vi "test_TxUDP.vi"() -> ()   [LabVIEW 2020]
uses:
  <instrlib>/AIM GmbH/_AIM 664/_controls/port_configuration.ctl
  <instrlib>/AIM GmbH/_AIM 664/_controls/port_speed.ctl
  <instrlib>/AIM GmbH/_AIM 664/_controls/comm_config_vl_tx.ctl
  <instrlib>/AIM GmbH/_AIM 664/_controls/comm_udp_tx.ctl
  <instrlib>/AIM GmbH/_AIM 664/helpers/EthFrameManagement/controls/arinc664_mac_src_info.ctl
  <instrlib>/AIM GmbH/_AIM 664/_controls/comm_computedMAC-IP.ctl
  <instrlib>/AIM GmbH/_AIM 664/bsp/Fdx Create Session (Tx-UDP Port-Oriented).vi
  <instrlib>/AIM GmbH/_AIM 664/bsp/Transmit/FdxCreateTxVL.vi
  <instrlib>/AIM GmbH/_AIM 664/bsp/Fdx Create UDP Port (TX-CommPort).vi
  <instrlib>/AIM GmbH/_AIM 664/bsp/Fdx Start (Tx).vi
  Global 1.vi
  <instrlib>/AIM GmbH/_AIM 664/bsp/Fdx Stop (Tx).vi
  <instrlib>/AIM GmbH/_AIM 664/AIM664LV.lvlib
  <instrlib>/AIM GmbH/_AIM 664/bsp/Fdx Create Session (Generic-Board).vi
  <instrlib>/AIM GmbH/_AIM 664/helpers/EthFrameManagement/EthFrameManagement.lvlib
panel:
  in  "index":i32
  out "Waveform Chart":u32(graph)
  out "CurrentIndex":u32
  out "IndexCycleCount":u32
  out "MsgCount":u32
  out "TxStatus":T1 {"TransmitMode" items=["FDX_TX_GENERIC", "FDX_TX_REPLAY", "FDX_TX_INDIVIDUAL"]; "TxStatus" items=["FDX_STAT_STOP", "FDX_STAT_RUN", "FDX_STAT_ERROR", "FDX_STAT_WAIT_F_TRIG"]}
  out "BytesWritten":u32
  in  "stop":bool
  out "IP configs":T2[](array[typedef]) {"MACsrc" format="%.0x"}
  out "Buf":u8[](array[numeric]) format="%.0x"
  in  "Buf Lenght":i32=512
  in  "VlTx":T3={"domainID"=1, "sideID"=1, "locationID"=1, "interfaceID"=1}
  in  "CommPort Config":T4[](array[typedef])=[{"PortType"=enum."FDX_UDP_SAMPLING", "partitionID"=1, "SubVlId"=1, "UdpSrcPort"=24, "UdpDstPort"=23, "SampleRateMs"=64.0, "UdpNumBufMessages"=1, "UdpMaxMessageSize"=512}]
  in  "VL Config":T5={"VlId"=60, "NumOfSubVl"=1, "rate ms [Bag]"=64, "domainID"=1, "sideID"=1, "locationID"=1, "interfaceID"=1, "NetSelect"=3, "Skew"=0, "MaxFrameLength"=1518, "FrameBufferSize"=0} {"NetSelect" items=["FDX_TX_FRAME_DLY_A"=0, "FDX_TX_FRAME_DLY_B"=1, "FDX_TX_FRAME_BOTH "=3, "FDX_TX_FRAME_ONLY_A"=4, "FDX_TX_FRAME_ONLY_B "=5]; "interfaceID" format="%.0b"}
  in  "PortMap":u32=1
  out "PortInitOut":T6 {"PortConfig" items=["FDX_SINGLE", "FDX_REDUNDANT"]}
  in  "port":u32
  in  "PortSpeed":T7[](array[typedef])=[0, 0] items=["FDX_100MBIT"=0, "FDX_10MBIT"=1, "FDX_1000MBIT"=5, "FDX_AUTO_100MBIT"=2, "FDX_AUTO_10MBIT"=3]
  in  "PortConfig":T8[](array[typedef])=[0, 0] items=["FDX_SINGLE", "FDX_REDUNDANT"]
  out "timed out":bool
  out "good link":bool
  out "error out":errorcluster
  in  "board":u32
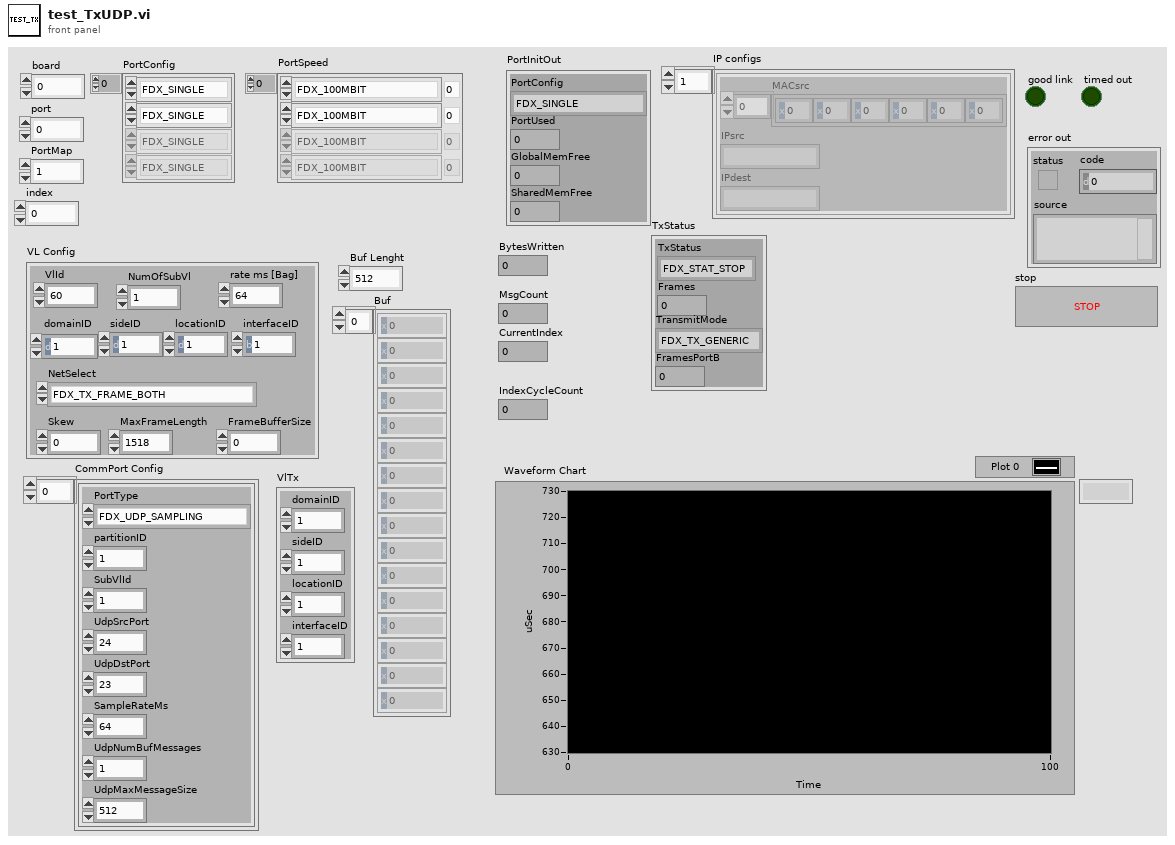
[diagram p1: front panel]
types:
  T1 = cluster{"TxStatus":u32, "Frames":u32, "TransmitMode":u32, "FramesPortB":u32}
  T2 = typedef "AIM664LV.lvlib/comm_computedMAC-IP.ctl" = cluster{"MACsrc":u8[], "IPsrc":string, "IPdest":string}
  T3 = typedef "EthFrameManagement.lvlib/arinc664_mac_src_info.ctl" = cluster{"domainID":u8, "sideID":u8, "locationID":u8, "interfaceID":u8}
  T4 = typedef "AIM664LV.lvlib/comm_udp_tx.ctl" = cluster{"PortType":enum16{"FDX_UDP_SAMPLING", "FDX_UDP_QUEUING"}, "partitionID":u8, "SubVlId":u8, "UdpSrcPort":u16, "UdpDstPort":u16, "SampleRateMs":dbl, "UdpNumBufMessages":u32, "UdpMaxMessageSize":u32}
  T5 = typedef "AIM664LV.lvlib/comm_config_vl_tx.ctl" = cluster{"VlId":u16, "NumOfSubVl":u16, "rate ms [Bag]":u32, "domainID":u8, "sideID":u8, "locationID":u8, "interfaceID":u8, "NetSelect":u32, "Skew":u32, "MaxFrameLength":u32, "FrameBufferSize":u32}
  T6 = cluster{"PortConfig":u32, "PortUsed":u32, "GlobalMemFree":u32, "SharedMemFree":u32}
  T7 = typedef "AIM664LV.lvlib/port_speed.ctl" = u32
  T8 = typedef "AIM664LV.lvlib/port_configuration.ctl" = u32
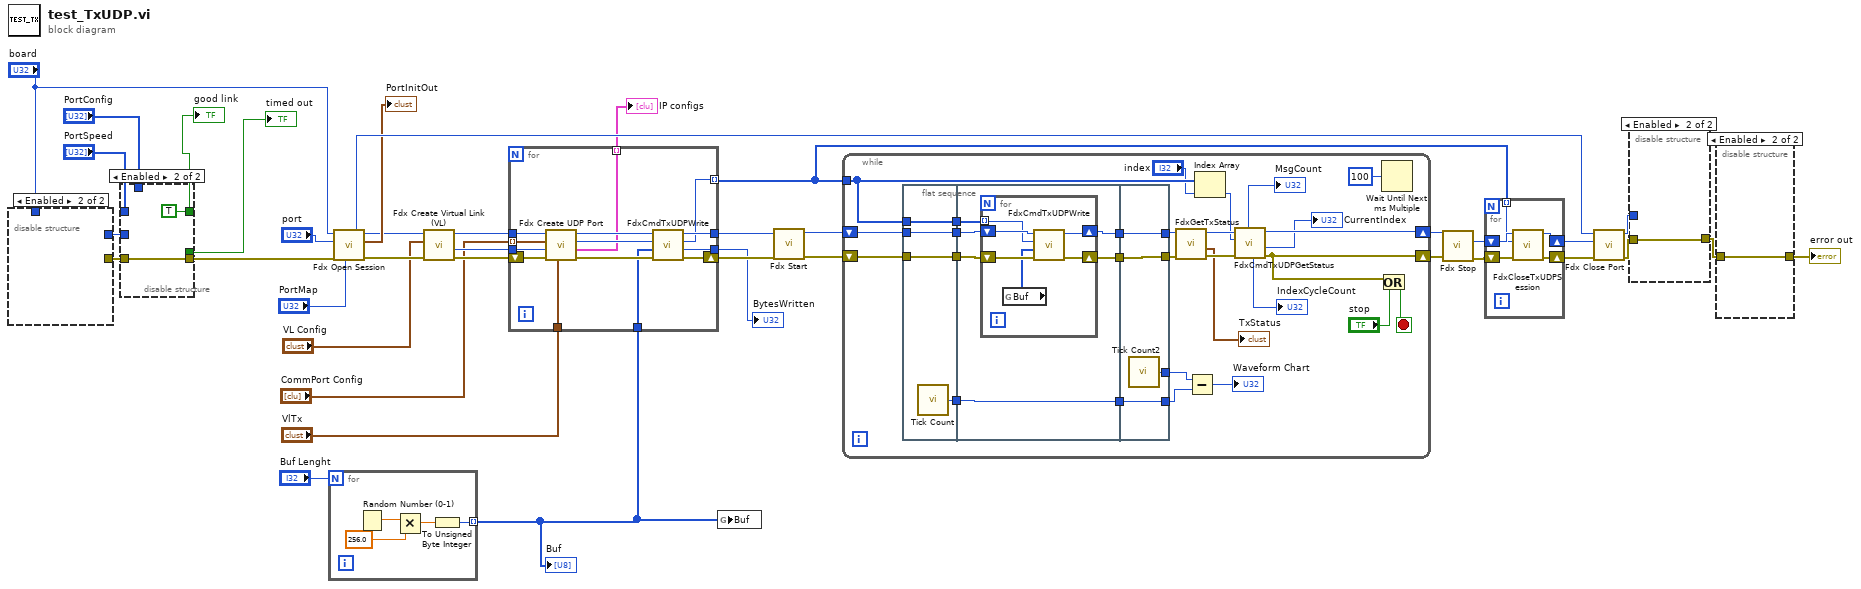
[diagram p0: block diagram]
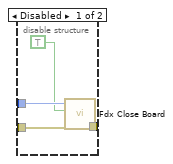
[diagram p2: hidden frame]
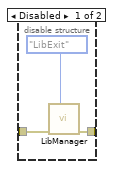
[diagram p3: hidden frame]
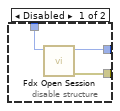
[diagram p4: hidden frame]
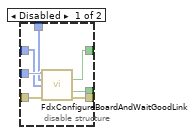
[diagram p5: hidden frame]
diagram:
  n1 = disable-structure shown="Enabled" {
    disable-tunnel: [w42 _] -> w39
    disable-tunnel: [w41 _] -> w38
    disable-tunnel: "board" -> [w40 _]
    frame Disabled {
      n2 = call-poly <instrlib>:"Fdx Open Session.vi"("board"=w40) -> ("error out"=w41:errorcluster, "InstrumentHandle_board out"=w42:u32)  [unwired: 8 in, 1 out]
    }
    frame Enabled {
    }
  }
  n3 = disable-structure shown="Enabled" {
    disable-tunnel: w39 -> [w49 _]
    disable-tunnel: w38 -> [w48 w51]
    disable-tunnel: [w47 TRUE ("good link")] -> w37
    disable-tunnel: [w46 _] -> w36
    disable-tunnel: "PortConfig" -> [w45 _]
    disable-tunnel: "PortSpeed" -> [w44 _]
    disable-tunnel: [w43 w51] -> w33
    frame Disabled {
      n4 = call <instrlib>:"FdxConfigureBoardAndWaitGoodLink.vi"("InstrumentHandle_board in"=w49, "PortConfig"=w45, "PortSpeed"=w44, "error in"=w48) -> ("good link"=w47:bool, "timed out"=w46:bool, "error out"=w43:errorcluster)  [unwired: 8 in, 1 out]
    }
    frame Enabled {
    }
  }
  "good link" <- w37
  "timed out" <- w36
  n5 = for {
    N: "Buf Lenght" -> [_]
    tunnel: [w52] -> w1 mode=indexing
    n6 = Random Number (0-1)() -> (number: 0 to 1=w55:dbl)
    n7 = Multiply(x=w55, y=256.0) -> (x*y=w53:dbl)
    n8 = To Unsigned Byte Integer(number=w53) -> (unsigned 8bit integer=w52:u8)
  }
  "Buf" <- w1
  n9 = call-poly <instrlib>:"Fdx Open Session.vi"("PortMap"="PortMap", "error in (no error)"=w33, "port"="port", "board"="board") -> ("error out"=w23:errorcluster, "PortInitOut"=→"PortInitOut":T6, "port handle out"=w22:u32, "InstrumentHandle_board out"=w28:u32)  [unwired: 3 in, 1 out]
  n10 = call-poly <instrlib>:"Fdx Create Virtual Link (VL).vi"("error in (no error)"=w23, "VL Config"="VL Config", "InstrumentHandle in"=w22) -> ("error out"=w18:errorcluster, "VlId"=w19:u16, "InstrumentHandle out"=w20:u32)  [unwired: 6 in]
  n11 = for {
    tunnel: w20 -> [w69]
    tunnel: w19 -> [w68]
    tunnel: "CommPort Config" -> [w66] mode=indexing
    tunnel: "VlTx" -> [w65]
    tunnel: [w61] -> w14 mode=indexing
    tunnel: [w59] -> w12
    tunnel: [w58] -> w9
    tunnel: [w57] -> w2 mode=indexing
    tunnel: w1 -> [w56]
    shift-right: [w60] -> w13
    shift-left: w18 -> [w67]
    n12 = call-poly <instrlib>:"Fdx Create UDP Port.vi"("VlTx"=w65, "error in"=w67, "VlId"=w68, "CommPort Config"=w66, "port handle in"=w69) -> ("error out"=w62:errorcluster, "computedAddresses"=w61:T2, "commPort handle out"=w63:u32, "port handle out"=w64:u32)  [unwired: 3 in]
    n13 = call <instrlib>:"FdxCmdTxUDPWrite.vi"("error in"=w62, "Data"=w56, "UdpHandle"=w63, "InstrumentHandle"=w64) -> ("error out"=w60:errorcluster, "BytesWritten"=w58:u32, "UdpHandleOut"=w57:u32, "InstrumentHandle"=w59:u32)  [unwired: 4 in]
  }
  "IP configs" <- w14
  "BytesWritten" <- w9
  n14 = global write "Global 1.vi" "Buf"(w1) -> ()
  n15 = call-poly <instrlib>:"Fdx Start.vi"("error in"=w13, "InstrumentHandle_port in"=w12) -> ("error out"=w11:errorcluster, "InstrumentHandle_port out"=w10:u32)  [unwired: 8 in]
  n16 = while {
    shift-right: [w91] -> w7
    shift-left: w10 -> [w85]
    shift-right: [w92] -> w8
    shift-left: w11 -> [w80]
    tunnel: w2 -> [w72]
    stop <- w95 stop-if-true
    n17 = flat-sequence {
      tunnel: [w101] -> w86
      tunnel: w85 -> [w101]
      tunnel: [w100] -> w82
      tunnel: w72 -> [w100]
      tunnel: [w99] -> w81
      tunnel: w80 -> [w99]
      tunnel: [w98] -> w78
      tunnel: w86 -> [w107]
      tunnel: [w106] -> w83
      tunnel: w82 -> [w105]
      tunnel: w81 -> [w104]
      tunnel: [w103] -> w79
      tunnel: w78 -> [w103]
      tunnel: [w102] -> w73
      tunnel: [w117] -> w84
      tunnel: w83 -> [w117]
      tunnel: [w116] -> w77
      tunnel: [w115] -> w76
      tunnel: w79 -> [w115]
      tunnel: [w114] -> w74
      tunnel: w73 -> [w114]
      frame #0 {
        n18 = call "Tick Count"() -> ("Tick Count(uSec)"=w98:u32)
      }
      frame #1 {
        n19 = for {
          tunnel: w105 -> [w111] mode=indexing
          shift-right: [w112] -> w106
          shift-left: w107 -> [w113]
          shift-right: [w108] -> w102
          shift-left: w104 -> [w110]
          n20 = global read "Global 1.vi" "Buf"() -> (w109:u8[])
          n21 = call <instrlib>:"FdxCmdTxUDPWrite.vi"("error in"=w110, "Data"=w109, "UdpHandle"=w111, "InstrumentHandle"=w113) -> ("error out"=w108:errorcluster, "InstrumentHandle"=w112:u32)  [unwired: 4 in, 2 out]
        }
      }
      frame #2 {
        n22 = call "Tick Count2"() -> ("Tick Count(uSec)"=w116:u32)
      }
    }
    n23 = call <instrlib>:"FdxGetTxStatus.vi"("error in"=w74, "InstrumentHandle_port"=w84) -> ("error out"=w94:errorcluster, "TxStatus"=→"TxStatus":T1, "InstrumentHandle_port"=w93:u32)  [unwired: 7 in]
    n24 = Subtract(x=w77, y=w76) -> (x-y=→"Waveform Chart":u32)
    n25 = Index Array(array=w72, index="index") -> (element=w71:u32)
    n26 = call <instrlib>:"FdxCmdTxUDPGetStatus.vi"("error in"=w94, "UdpHandle"=w71, "InstrumentHandle"=w93) -> ("error out"=w92:errorcluster, "CurrentIndex"=→"CurrentIndex":u32, "InstrumentHandle"=w91:u32, "IndexCycleCount"=→"IndexCycleCount":u32, "MsgCount"=→"MsgCount":u32)  [unwired: 3 in, 1 out]
    n27 = Or(x=w92, y="stop") -> (x .or. y?=w95:bool)
    n28 = Wait Until Next ms Multiple(millisecond multiple=u32 100) -> ()  [unwired: 1 out]
  }
  n29 = call-poly <instrlib>:"Fdx Stop.vi"("error in"=w8, "InstrumentHandle_port in"=w7) -> ("error out"=w6:errorcluster, "InstrumentHandle_port out"=w3:u32)  [unwired: 8 in]
  n30 = for {
    tunnel: w2 -> [w118] mode=indexing
    shift-right: [w121] -> w5
    shift-left: w6 -> [w122]
    shift-right: [w120] -> w4
    shift-left: w3 -> [w119]
    n31 = call <instrlib>:"FdxCloseTxUDPSession.vi"("error in"=w122, "UdpHandle"=w118, "InstrumentHandle"=w119) -> ("error out"=w121:errorcluster, "InstrumentHandle"=w120:u32)  [unwired: 7 in]
  }
  n32 = call <instrlib>:"Fdx Close Port.vi"("error in"=w5, "InstrumentHandle_port in"=w4, "InstrumentHandle_board in"=w28) -> ("error out"=w30:errorcluster, "InstrumentHandle_board out"=w29:u32)  [unwired: 7 in]
  n33 = disable-structure shown="Enabled" {
    disable-tunnel: w30 -> [w126 w127]
    disable-tunnel: w29 -> [w125 _]
    disable-tunnel: [w123 w127] -> w25
    frame Disabled {
      n34 = call <instrlib>:"Fdx Close Board.vi"("error in"=w126, "Force Board Release (F)"=TRUE ("Close reference to library?"), "InstrumentHandle_board in"=w125) -> ("error out"=w123:errorcluster)  [unwired: 8 in]
    }
    frame Enabled {
    }
  }
  n35 = disable-structure shown="Enabled" {
    disable-tunnel: w25 -> [w129 w131]
    disable-tunnel: [w128 w131] -> w24
    frame Disabled {
      n36 = call <instrlib>:"LibManager.vi"("action"=enum16{"LibInit", "LibExit"}."LibExit", "error in (no error)"=w129) -> ("error out"=w128:errorcluster)  [unwired: 7 in, 2 out]
    }
    frame Enabled {
    }
  }
  "error out" <- w24
